vi "ErrorCheckHWI.vi"(8 "error in (no error)":errorcluster, 11 "Arduino in":refnum<class "Arduino.lvclass">) -> (0 "error out":errorcluster, 3 "Arduino out":refnum<class "Arduino.lvclass">)   [LabVIEW 2013, in "Arduino.lvclass"]
uses:
  Arduino.lvclass
  Device/Device.lvclass
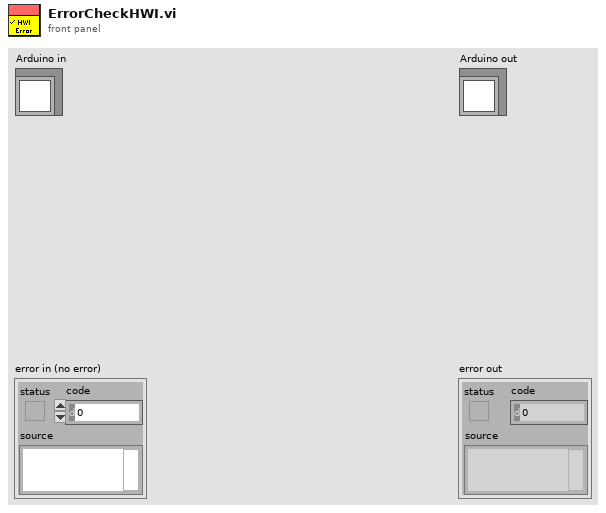
[diagram p1: front panel]
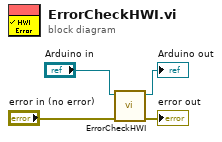
[diagram p0: block diagram]
diagram:
  n1 = call-parent "ErrorCheckHWI.vi"("error in (no error)"="error in (no error)", "Device in"="Arduino in") -> ("error out"=→"error out":errorcluster, "Device out"=→"Arduino out":refnum<class "Arduino.lvclass">)  [unwired: 8 in]
